vi "Read Waveform Measurement Statistics.vi"(8 "error in (no error)":errorcluster, 10 "Measurement Number (0: Measurement 1)":i32(ring) items=["Measurement 1", "Measurement 2", "Measurement 3", "Measurement 4"], 11 "VISA resource name":refnum<visa-resource-name>) -> (0 "error out":errorcluster, 1 "Minimum Value":dbl, 2 "Maximum Value":dbl, 3 "VISA resource name out":refnum<visa-resource-name>, 4 "Standard Deviation":dbl, 5 "Mean Value":dbl)   [LabVIEW 2009, in "Tektronix DPO MSO 2000 4000 Series.lvlib"]
doc: "Returns the statistical values for the measurement channel you specified since the last statistical reset."
uses:
  <instrlib>/Tektronix DPO MSO 2000 4000 Series/Tektronix DPO MSO 2000 4000 Series.lvlib
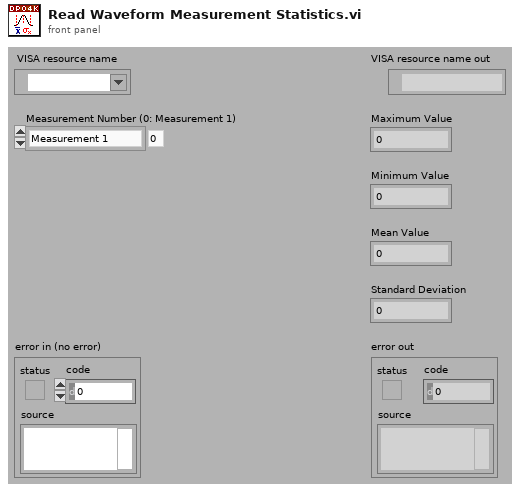
[diagram p1: front panel]
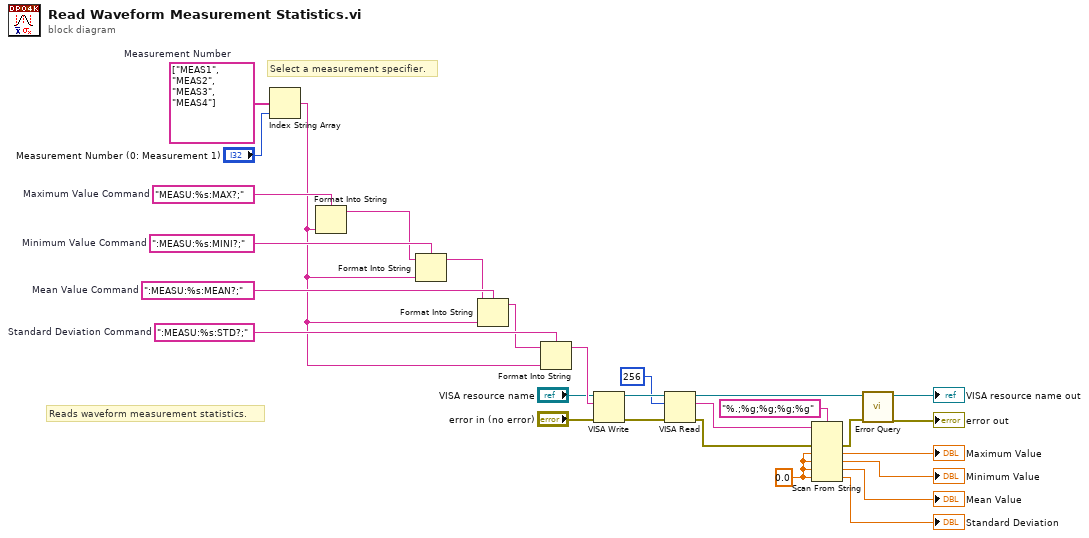
[diagram p0: block diagram]
diagram:
  w7 = 0.0 ("default value 1")
  w16 = string[] ["MEAS1", "MEAS2", "MEAS3", "MEAS4"]  # Measurement Number
  w25 = ":MEASU:%s:STD?;"  # Standard Deviation Command
  w26 = ":MEASU:%s:MINI?;"  # Minimum Value Command
  w27 = ":MEASU:%s:MEAN?;"  # Mean Value Command
  w28 = "MEASU:%s:MAX?;"  # Maximum Value Command
  # "Select a measurement specifier."
  # "Reads waveform measurement statistics."
  n1 = Index String Array(1:"Measurement Number (0: Measurement 1)", 2:w16) -> (0:w14:string)  [unwired: 1 in]
  n2 = Format Into String(format string=w28, w14) -> (resulting string=w18:string)  [unwired: 2 in, 1 out]
  n3 = Format Into String(format string=w26, initial string=w18, w14) -> (resulting string=w19:string)  [unwired: 1 in, 1 out]
  n4 = Format Into String(format string=w27, initial string=w19, w14) -> (resulting string=w17:string)  [unwired: 1 in, 1 out]
  n5 = Format Into String(format string=w25, initial string=w17, w14) -> (resulting string=w24:string)  [unwired: 1 in, 1 out]
  n6 = VISA Write(VISA resource name="VISA resource name", write buffer=w24, error in (no error)="error in (no error)") -> (VISA resource name out=w13:refnum<visa-resource-name>, error out=w12:errorcluster)  [unwired: 1 out]
  n7 = VISA Read(VISA resource name=w13, byte count=u32 256, error in (no error)=w12) -> (VISA resource name out=w10:refnum<visa-resource-name>, read buffer=w8:string, error out=w2:errorcluster)  [unwired: 1 out]
  n8 = Scan From String(format string="%.;%g;%g;%g;%g", input string=w8, error in=w2, default 1=w7, default 2=w7, default 3=w7, default 4=w7) -> (error out=w1:errorcluster, output 1=→"Maximum Value":dbl, output 2=→"Minimum Value":dbl, output 3=→"Mean Value":dbl, output 4=→"Standard Deviation":dbl)  [unwired: 1 in, 2 out]
  n9 = call <instrlib>:"Error Query.vi"("error in (no error)"=w1, "VISA resource name"=w10) -> ("error out"=→"error out":errorcluster, "VISA resource name out"=→"VISA resource name out":refnum<visa-resource-name>)  [unwired: 6 in, 2 out]
